vi "AKD Enact Move.vi"(6 "Next MT?":bool, 7 "Motion type":enum16{"Rel", "Abs"}(ring)=enum."Abs", 8 "error in (no error)":errorcluster, 9 "Motion Task parameters":T1, 10 "MT ID":u16, 11 "TCP Refnum in":refnum<k5>) -> (0 "error out":errorcluster, 3 "TCP Refnum":refnum<k5>)   [LabVIEW 2009]
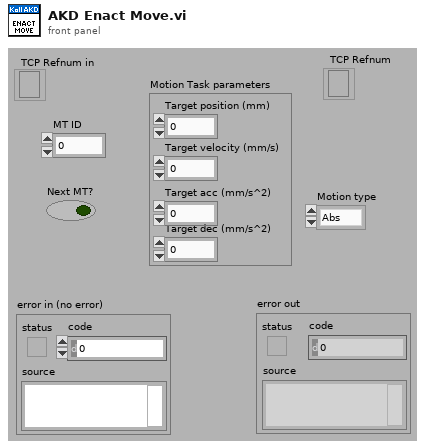
[diagram p1: front panel]
types:
  T1 = cluster{"Target position (mm)":sgl, "Target velocity (mm/s)":sgl, "Target acc (mm/s^2)":sgl, "Target dec (mm/s^2)":sgl}
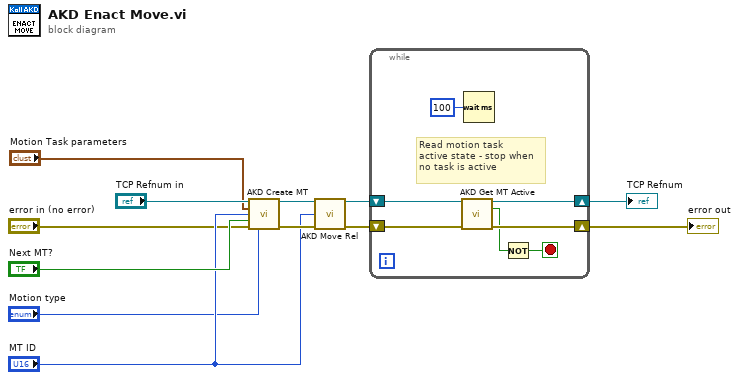
[diagram p0: block diagram]
diagram:
  n1 = call "AKD Create MT.vi"("TCP Refnum in"="TCP Refnum in", "Motion Task parameters"="Motion Task parameters", "Task no"="MT ID", "Next MT?"="Next MT?", "error in"="error in (no error)", "Motion type"="Motion type") -> ("TCP Refnum out"=w8:refnum<k5>, "error out"=w9:errorcluster)  [unwired: 8 in]
  n2 = call "AKD Move Rel.vi"("TCP Refnum in"=w8, "MT ID"="MT ID", "error in"=w9) -> ("TCP Refnum out"=w10:refnum<k5>, "error out"=w11:errorcluster)  [unwired: 11 in]
  n3 = while {
    shift-right: [w18] -> w3
    shift-left: w10 -> [w15]
    shift-right: [w19] -> w4
    shift-left: w11 -> [w14]
    stop <- w16 stop-if-true
    # "Read motion task\nactive state - stop when\nno task is active"
    n4 = call "AKD Get MT Active.vi"("TCP Refnum in"=w15, "error in"=w14) -> ("TCP Refnum out"=w18:refnum<k5>, "MT active?"=w17:bool, "error out"=w19:errorcluster)  [unwired: 10 in, 1 out]
    n5 = Wait (ms)(milliseconds to wait=u32 100) -> ()  [unwired: 1 out]
    n6 = Not(x=w17) -> (.not. x?=w16:bool)
  }
  "error out" <- w4
  "TCP Refnum" <- w3
